vi "Initialize Addon.vi"(8 "error in (no error)":errorcluster, 10 "Diagnostics Basic Configuraiton":T2, 11 "Device Item Ref in":T1 format="%.0x") -> (0 "error out":errorcluster, 3 "Device Item Ref out":T1=18446744073709551615 format="%.0x")   [LabVIEW 2015, in "Diagnostics Addon System Explorer.lvlib"]
uses:
  Diagnostics Addon System Explorer.lvlib
  Types/Base Configuration.ctl
  Shared/Types/CAN Interface.ctl
  Shared/Types/Diagnostic Protocols.ctl
  <vilib>/NI Veristand/Custom Device API/Custom Device Item Ref.ctl
  <vilib>/NI Veristand/Custom Device Tools/Custom Device Utility Library/NI VeriStand - Search for Item by Name.vi
  <vilib>/NI Veristand/Custom Device Tools/Custom Device Utility Library/NI VeriStand - Search for Item by GUID.vi
  Shared/SubVIs/GUID Lookup.vi
  Shared/Diagnostics Addon Shared.lvlib
  <vilib>/NI Veristand/Custom Device Tools/Custom Device Utility Library/Custom Device Utility Library.lvlib
  <vilib>/NI Veristand/Custom Device API/Custom Device API.lvlib
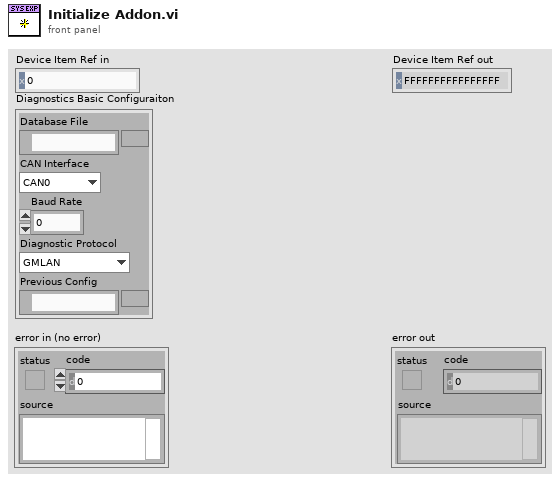
[diagram p1: front panel]
types:
  T1 = typedef "Custom Device API.lvlib/Custom Device Item Ref.ctl" = u64
  T2 = typedef "Diagnostics Addon System Explorer.lvlib/Base Configuration.ctl" = cluster{"Database File":path, "CAN Interface":T3, "Baud Rate":u32, "Diagnostic Protocol":T4, "Previous Config":path}
  T3 = typedef "Diagnostics Addon Shared.lvlib/CAN Interface.ctl" = enum16{"CAN0", "CAN1", "CAN2", "CAN3", "CAN4", "CAN5", "CAN6", "CAN7", "CAN8", "CAN9", "CAN10", "CAN11", "CAN12", "CAN13", "CAN14", "CAN15", "CAN16", "CAN17", "CAN18", "CAN19", "CAN20", "CAN21", "CAN22", "CAN23", "CAN24", "CAN25", "CAN26", "CAN27", "CAN28", "CAN29", "CAN30", "CAN31", "CAN32", "CAN33", "CAN34", "CAN35", "CAN36", "CAN37", "CAN38", "CAN39", "CAN40", "CAN41", "CAN42", "CAN43", "CAN44", "CAN45", "CAN46", "CAN47", "CAN48", "CAN49", "CAN50", "CAN51", "CAN52", "CAN53", "CAN54", "CAN55", "CAN56", "CAN57", "CAN58", "CAN59", "CAN60", "CAN61", "CAN62", "CAN63", "CAN 256 (Virtual)", "CAN 257 (Virtual)"}
  T4 = typedef "Diagnostics Addon Shared.lvlib/Diagnostic Protocols.ctl" = enum16{"GMLAN", "KWP-2000", "UDS"}
  T5 = typedef "Diagnostics Addon System Explorer.lvlib/Exported Configuration.ctl" = cluster{"Name":string, "Description":string, "Diagnostics Basic Configuraiton":T6, "DIDs":T9, "Input PIDs":T9, "Output PIDs":T9, "DPIDs":T12, "DTC":T16, "NI 986x Support":T19, "Commands":T20, "Status":T21, "IO Controls":T22, "Routines":T25, "Output Memory":T9, "Input Memory":T9}
  T6 = typedef "Diagnostics Addon Shared.lvlib/CAN Configuration.ctl" = cluster{"Database File":path, "CAN Interface":T3, "Baud Rate":u32, "Diagnostic Protocol":T4, "Transport Protocol":T7, "Transmit ID":u32, "Receive ID":u32, "Transmit Extension":u8, "Receive Extension":u8, "Receive UUDT ID":u32, "Enable Stream":bool, "VW TP Channel ID":u32, "Security":T8, "Fill Frame":bool, "Fill Byte":u8, "Termination":bool}
  T7 = typedef "Diagnostics Addon Shared.lvlib/Transport Protocols.ctl" = enum16{"ISO TP - Normal Mode", "ISO TP - Mixed Mode", "VW TP 2.0", "Diagnostics on IP"}
  T8 = typedef "Diagnostics Addon Shared.lvlib/Security.ctl" = cluster{"Source DLL Path":path, "Security Level":u8, "Target DLL Path":path}
  T9 = typedef "Diagnostics Addon System Explorer.lvlib/Exported Frames Cluster.ctl" = cluster{"Description":string, "Frames":T10[]}
  T10 = typedef "Diagnostics Addon Shared.lvlib/Frame Parameters.ctl" = cluster{"Name":string, "Description":string, "ID":u16, "Signals":T11[]}
  T11 = typedef "Diagnostics Addon Shared.lvlib/Signal Parameters.ctl" = cluster{"Start Bit":u8, "Length":u8, "Scaling Factor":dbl, "Scaling Offset":dbl, "Minimum":dbl, "Maximum":dbl, "Data Type":u32, "Byte Order":u32, "Default Value":dbl, "Name":string, "Units":string, "Description":string}
  T12 = typedef "Diagnostics Addon System Explorer.lvlib/Exported DPIDs Cluster.ctl" = cluster{"Description":string, "DPIDs":T13[]}
  T13 = typedef "Diagnostics Addon System Explorer.lvlib/Exported DPID Parameters.ctl" = cluster{"Name":string, "Description":string, "DPID":T14}
  T14 = typedef "Diagnostics Addon Shared.lvlib/DPID Parameters.ctl" = cluster{"DPID ID":u8, "Speed":T15, "PIDs":u16[]}
  T15 = typedef "Diagnostics Addon Shared.lvlib/DPID Periodic Rate.ctl" = enum16{"Slow", "Medium", "Fast"}
  T16 = typedef "Diagnostics Addon System Explorer.lvlib/Exported DTC Cluster.ctl" = cluster{"Description":string, "DTC descriptor":T17, "DTCControl":T18}
  T17 = typedef "Diagnostics Addon Shared.lvlib/DTC Descriptor.ctl" = cluster{"DTC Byte Length":i32, "Status Byte Length":i32, "Add Data Byte Length":i32, "Byte Order":enum16{"Motorola", "Intel"}}
  T18 = typedef "Diagnostics Addon System Explorer.lvlib/Exported DTC Control Cluster.ctl" = cluster{"Description":string, "Signals":T11[]}
  T19 = typedef "Diagnostics Addon System Explorer.lvlib/Exported 986x Support.ctl" = cluster{"Enable 986x":bool, "RIO Device":u16, "Bitfile":path}
  T20 = typedef "Diagnostics Addon System Explorer.lvlib/Exported Command Cluster.ctl" = cluster{"Description":string}
  T21 = typedef "Diagnostics Addon System Explorer.lvlib/Exported Status Cluster.ctl" = cluster{"Description":string}
  T22 = typedef "Diagnostics Addon System Explorer.lvlib/Exported IO Control Cluster.ctl" = cluster{"Description":string, "IO Control Array":T23[]}
  T23 = typedef "Diagnostics Addon Shared.lvlib/IO Control Parameters.ctl" = cluster{"Name":string, "Description":string, "ID":u16, "Signals":T24}
  T24 = typedef "Diagnostics Addon Shared.lvlib/Command Response Signals.ctl" = cluster{"Cmd":T11[], "Response":T11[]}
  T25 = typedef "Diagnostics Addon System Explorer.lvlib/Exported Routines Cluster.ctl" = cluster{"Description":string, "Routine Array":T26[]}
  T26 = typedef "Diagnostics Addon Shared.lvlib/Routine Paramaters.ctl" = cluster{"Name":string, "Description":string, "ID":u16, "Start Parameters":T24, "Request Parameters":T24, "Stop Parameters":T24}
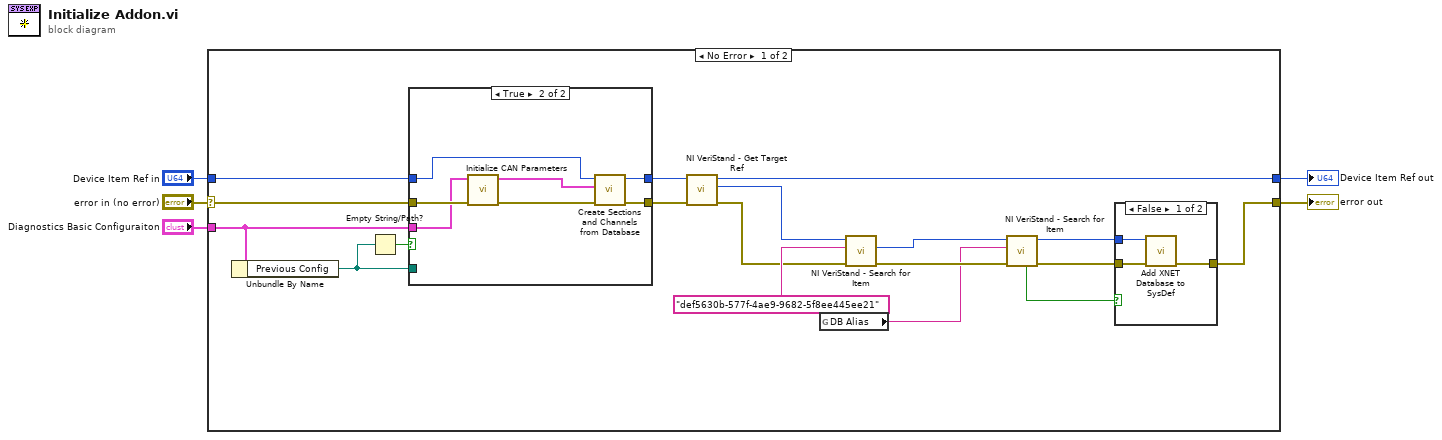
[diagram p0: block diagram]
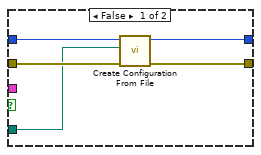
[diagram p3: hidden frame]
diagram:
  n1 = case shown="No Error" "error in (no error)" {
    selector: "error in (no error)" -> [w23 w40]
    tunnel: "Diagnostics Basic Configuraiton" -> [w21 _]
    tunnel: "Device Item Ref in" -> [w22 w41]
    tunnel: [w8 w41] -> w1
    tunnel: [w18 w40] -> w2
    frame No Error {
      n2 = Unbundle By Name(w21) -> ("Previous Config"=w19:path)
      n3 = Empty String/Path?(string/path=w19) -> (empty?=w20:bool)
      n4 = case shown="True" w20 {
        tunnel: [w31 w39] -> w10
        tunnel: [w30 w38] -> w13
        tunnel: w23 -> [w32 w37]
        tunnel: w22 -> [w29 w35]
        tunnel: w21 -> [_ w34]
        tunnel: w19 -> [w28 _]
        frame False {
          n5 = call "Create Configuration From File.vi"("error in (no error)"=w32, "Path in"=w28, "Device Item Ref in"=w29) -> ("error out"=w30:errorcluster, "Ref out"=w31:T1)  [unwired: 7 in]
        }
        frame True {
          n6 = call "Initialize CAN Parameters.vi"("error in (no error)"=w37, "Diagnostics Basic Configuraiton"=w34) -> ("error out"=w36:errorcluster, "Configuration"=w33:T5)  [unwired: 8 in]
          n7 = call "Create Sections and Channels from Database.vi"("error in (no error)"=w36, "Configuration"=w33, "Device Item Ref out in"=w35) -> ("error out"=w38:errorcluster, "Device Item Ref out out"=w39:T1)  [unwired: 7 in]
        }
      }
      n8 = call <vilib>:"NI VeriStand - Get Target Ref.vi"("error in"=w13, "Item Ref in"=w10) -> ("error out"=w14:errorcluster, "Target Ref"=w12:T1, "Item Ref out"=w8:T1)  [unwired: 6 in, 1 out]
      n9 = global read "GUID Lookup.vi" "DB Alias"() -> (w11:string)
      n10 = call-poly <vilib>:"NI VeriStand - Search for Item.vi"("error in"=w14, "Item GUID"="def5630b-577f-4ae9-9682-5f8ee445ee21" ("string"), "Section Ref in"=w12) -> ("error out"=w15:errorcluster, "Item Ref"=w16:T1)  [unwired: 5 in, 2 out]
      n11 = call-poly <vilib>:"NI VeriStand - Search for Item.vi"("error in"=w15, "Item Name"=w11, "Section Ref in"=w16) -> ("error out"=w9:errorcluster, "Section Ref out"=w7:T1, "Found"=w6:bool)  [unwired: 5 in, 1 out]
      n12 = case shown="False" w6 {
        tunnel: [w26 w27] -> w18
        tunnel: w9 -> [w25 w27]
        tunnel: w7 -> [w24 _]
        frame False {
          n13 = call "Add XNET Database to SysDef.vi"("error in (no error)"=w25, "Databases Section Ref"=w24) -> ("error out"=w26:errorcluster)  [unwired: 9 in]
        }
        frame True {
        }
      }
    }
    frame Error {
    }
  }
  "error out" <- w2
  "Device Item Ref out" <- w1
